vi "RPwithGaGe.vi"(8 "Error In":errorcluster, 10 "Server port":u16=1002, 11 "Server address":string="192.168.1.100") -> (0 "Error Out":errorcluster)   [LabVIEW 2015]
uses:
  Libraries/Red Pitaya/RP Command.ctl
  Libraries/Utilities/Controls/Integrate channel.ctl
  Libraries/GaGe-DAQ/GaGe Digitizer/GaGe Digitizer.lvclass
  Libraries/Red Pitaya/Mode.ctl
  Libraries/Red Pitaya/Red Pitaya Parameters.ctl
panel:
  out "Idot detected":bool
  out "Magnet current":waveform(dbl)(graph)
  in  "Controls":enum32{"Basic", "Advanced"}(tab)
  in  "Idot \ncalibration":dbl=-137722.0
  in  "Parameters":T1={"Ranges"=[1.12291, 20.0], "Output frequency 1"=50000.0, "Output frequency 2"=50000.0, "Trigger offset"=-2000000, "Post-trigger samples"=5767168, "Desimation rate"=64} {"Post-trigger samples" format="0x%x (%d)"; "Trigger offset" format="0x%x (%d)"; "Output frequency 2" format="%#_6p"; "Output frequency 1" format="%#_6p"; "Ranges" format="%#_12g"}
  out "CPU Temperature":dbl(slide)=48.847186279148 scale=0.0..100.0
  out "Current min/max":cluster{"Max":dbl, "Min":dbl}
  in  "Offset duration":dbl=0.95
  in  "Ch to \nintegrate":i32
  in  "Trigger pos acuracy":i32=2
  in  "Signal bits":i32=16
  in  "Read Temperature":bool=TRUE
  in  "Read trigger":bool=TRUE
  in  "Start server":bool
  in  "FPGA Logic":enum16{"Digitizer", "Fast Digitizer"}(ring)
  in  "Auto-save file":bool=TRUE
  in  "Samples to read":u64=67108864 format="0x%x (%d)"
  in  "Record":bool
  out "Server  output":string
  out "Temperature Chart":dbl(graph)=48.847186279148
  out "bytes written":i32=8
  in  "Status":bool
  out "Status response":u32=1
  out "element":u32
  in  "Status offset":u64=8 format="%x"
  out "Record start pos":u32=1
  out "x-y":u32=4294967295
  out "Phase increment 2":u64=1717987
  out "Phase increment 1":u64=1717987
  in  "Process Stop Button":bool
  in  "Read":bool
  in  "Read subset":bool
  out "Data File  Path":path
  out "Trigger state":bool
  in  "Trigger":bool
  in  "Arm":bool
  out "Phase  Graph":u32[](graph)
  in  "Mode":T2=enum."Digitizer"
  out "Waveform Graph":waveform(sgl)[](graph)
  in  "Stop Server":bool
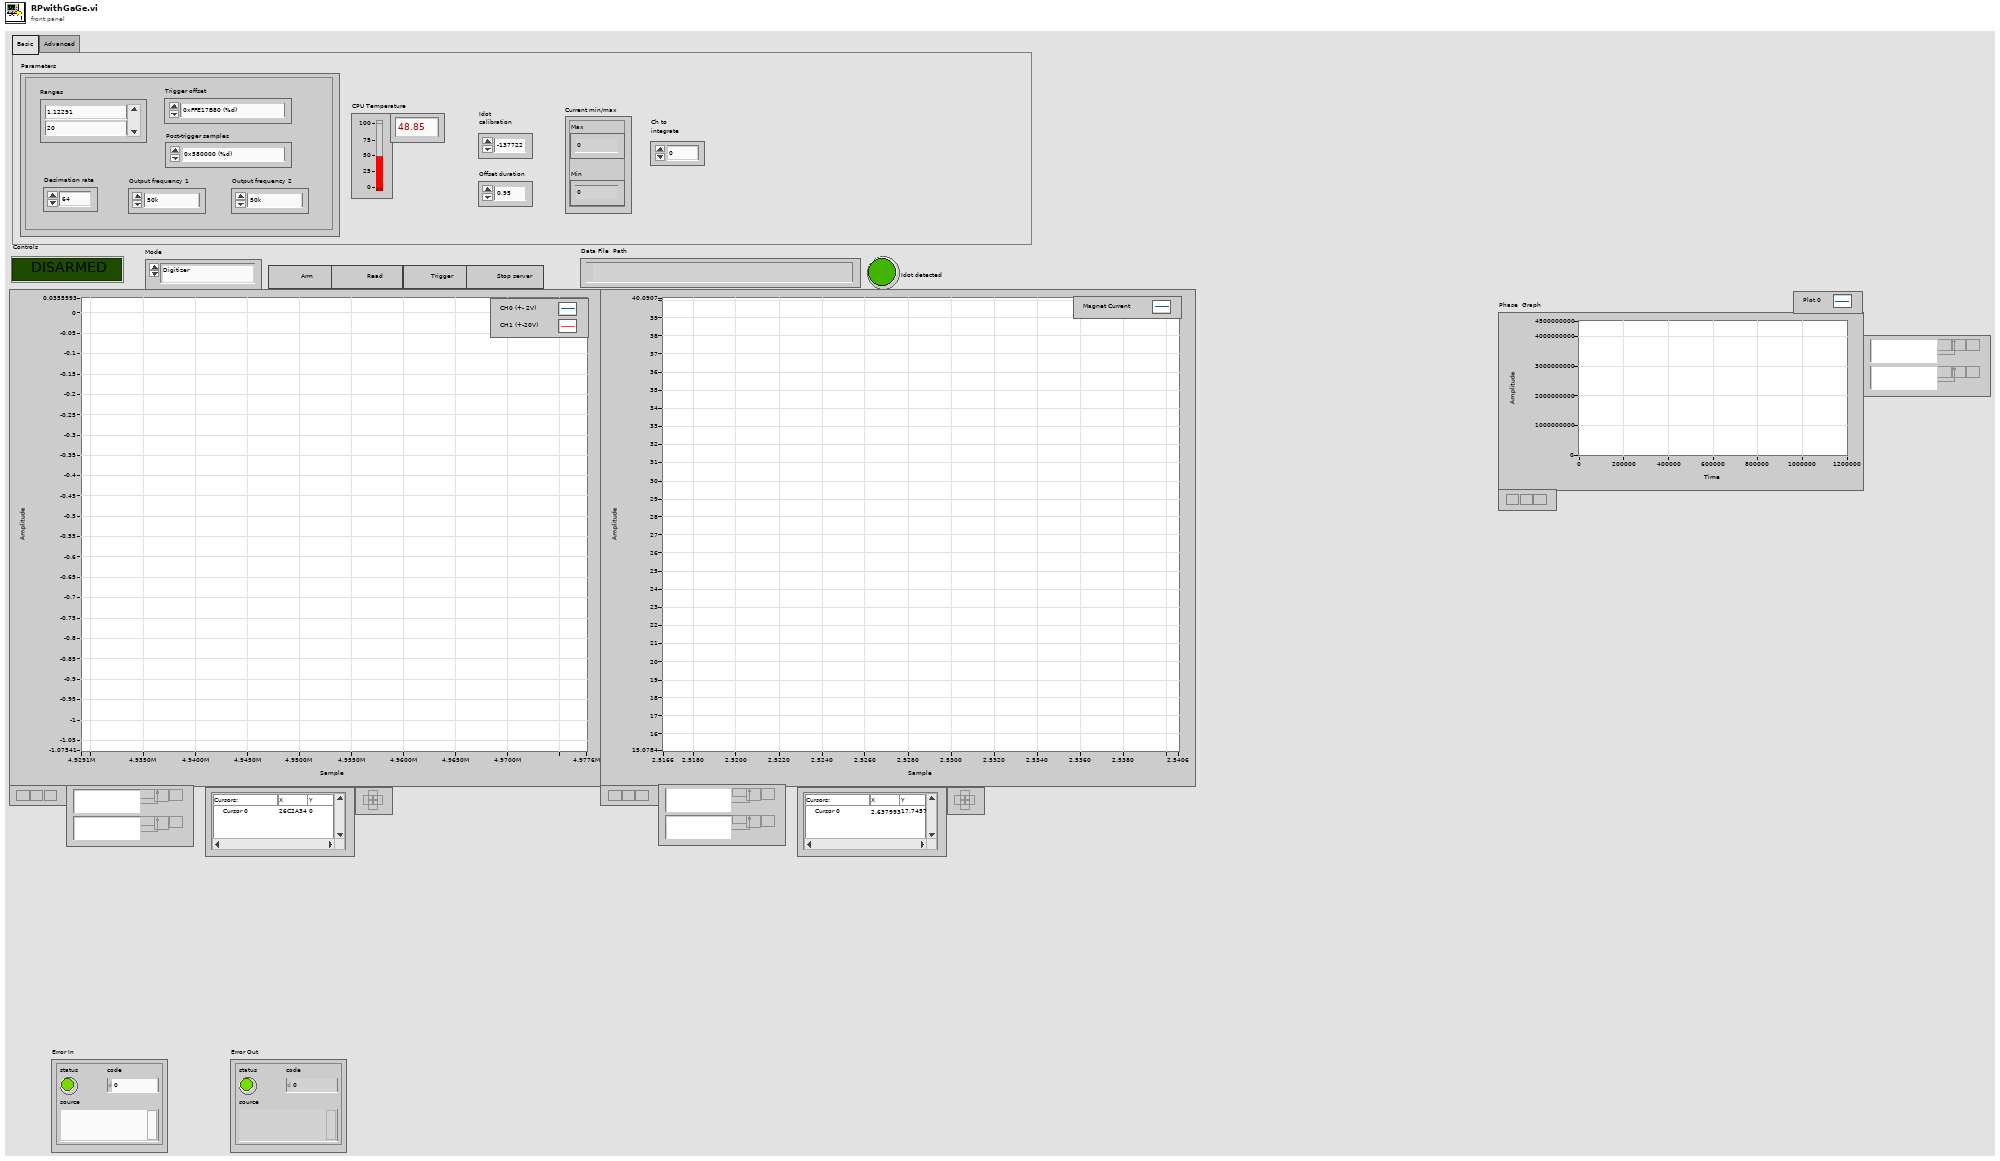
[diagram p1: front panel]
types:
  T1 = typedef "Red Pitaya Parameters.ctl" = cluster{"Ranges":dbl[], "Output frequency 1":dbl, "Output frequency 2":dbl, "Trigger offset":i32, "Post-trigger samples":u64, "Desimation rate":u64}
  T2 = typedef "Mode.ctl" = enum16{"Filter", "Lockin test", "Snapshot test", "Digitizer"}
  T3 = typedef "RP Command.ctl" = enum16{"Set frequency", "Arm and get data", "Stop server", "Get status", "Get temperature", "Set decimation", "Arm", "Software trigger", "Get whole buffer", "Get chunk", "System call", "Get config", "Set config", "Read FIFO", "Play pattern", "Set frequency batch"}
  T4 = enum16{"open", "open or create", "create or replace", "create", "open (read-only)"}
  T5 = typedef "Integrate channel.ctl" = cluster{"Channel":string, "Output name":string, "Factor":dbl, "Start time":dbl, "Duration":dbl}
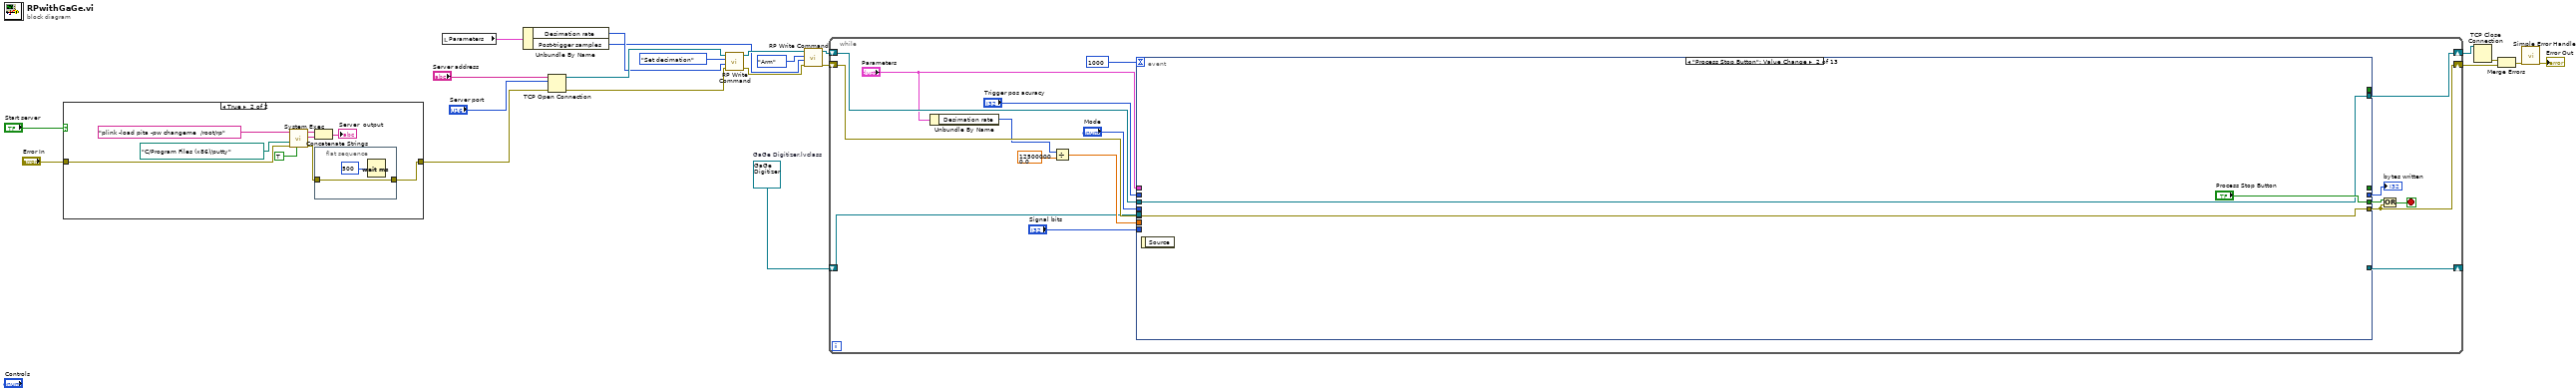
[diagram p0: block diagram]
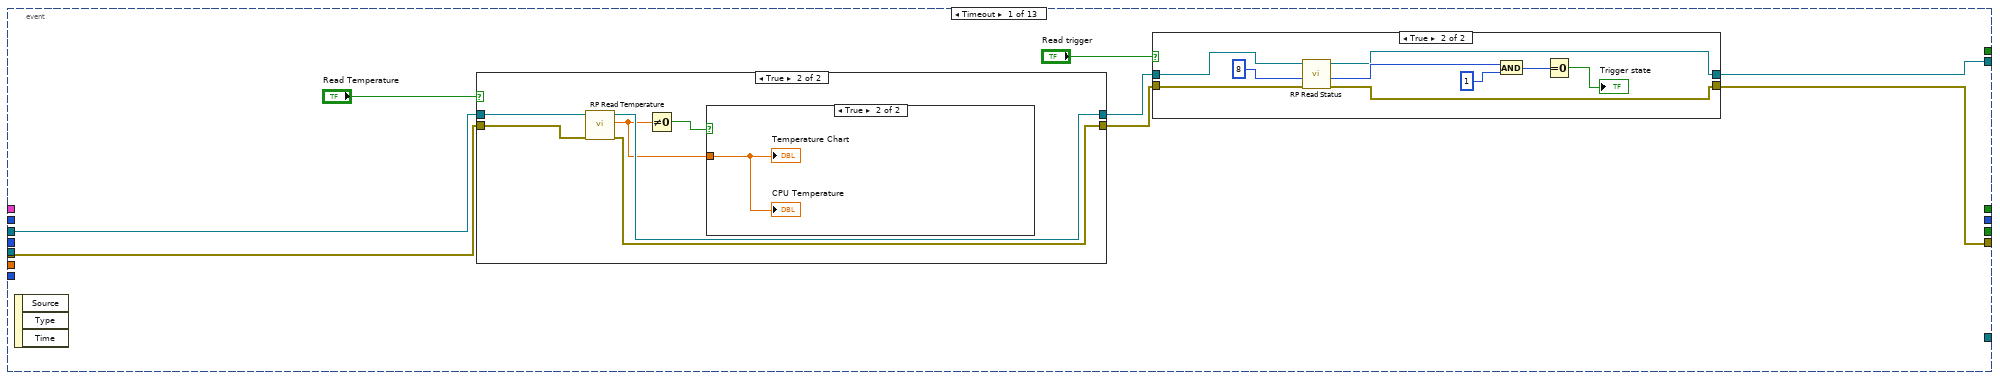
[diagram p3: hidden frame]
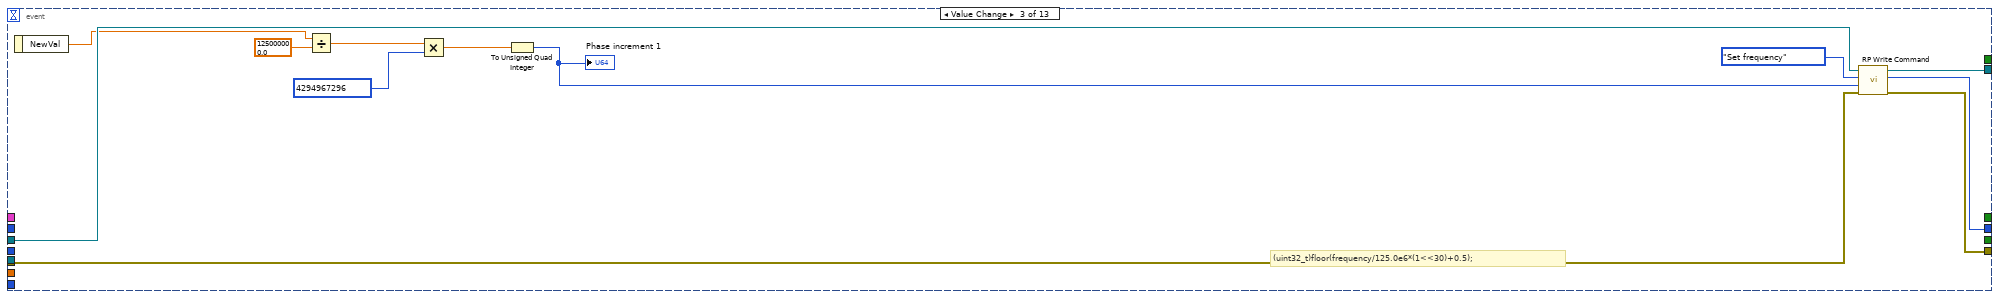
[diagram p7: hidden frame]
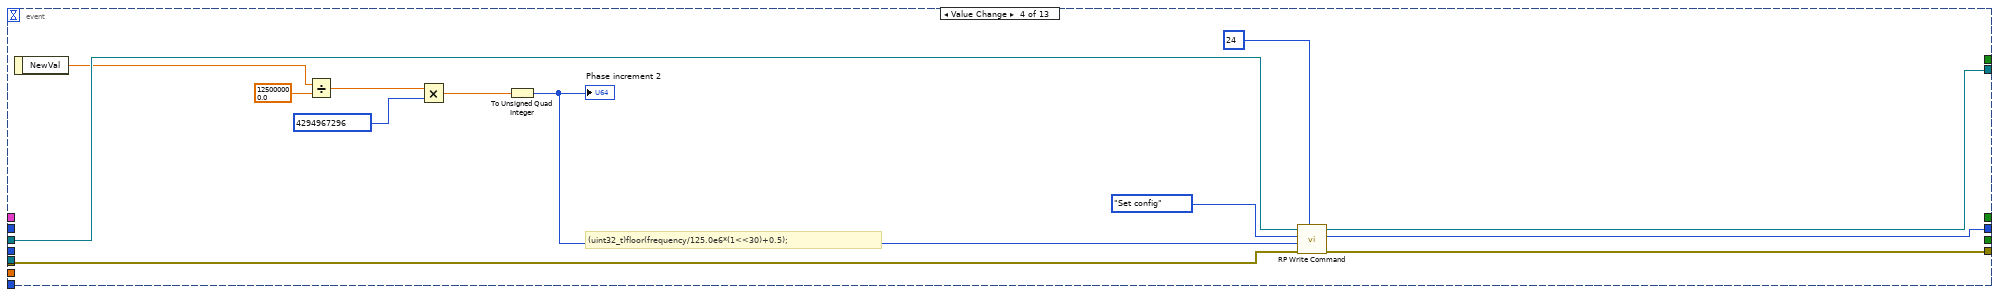
[diagram p8: hidden frame]
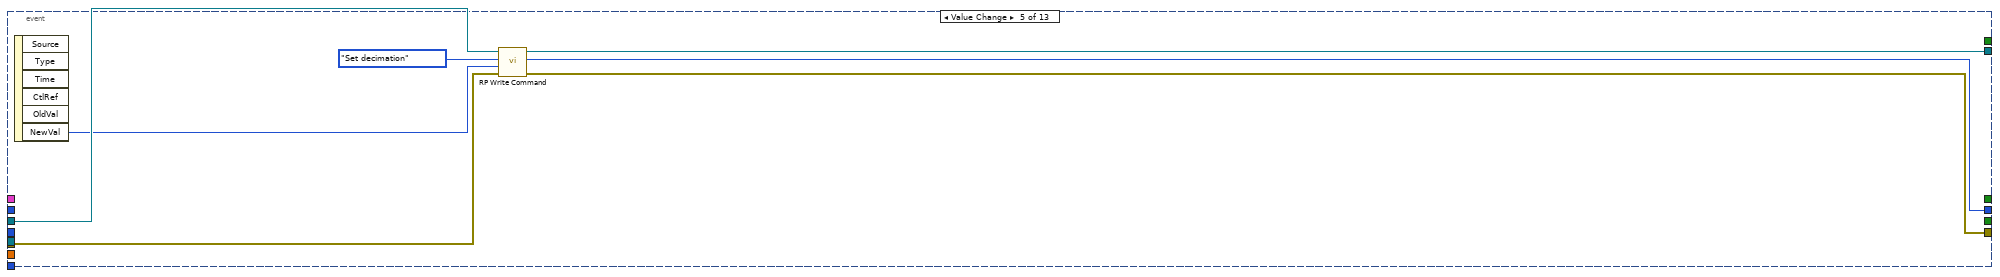
[diagram p9: hidden frame]
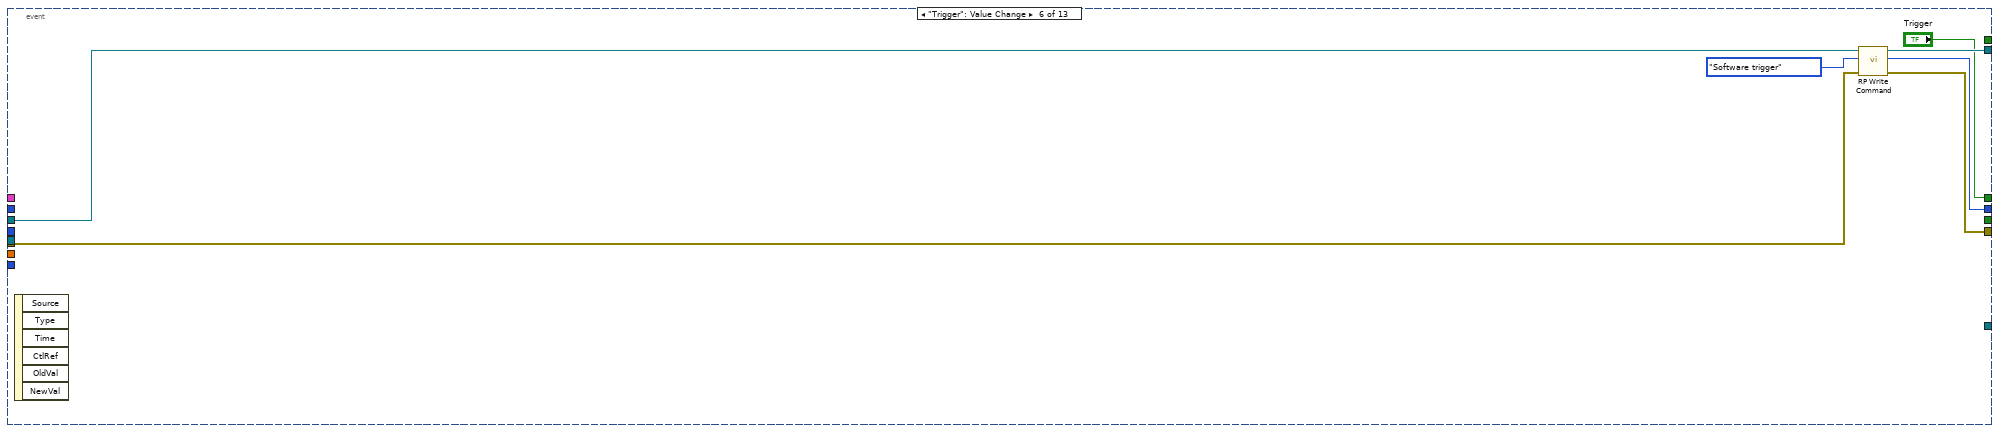
[diagram p10: hidden frame]
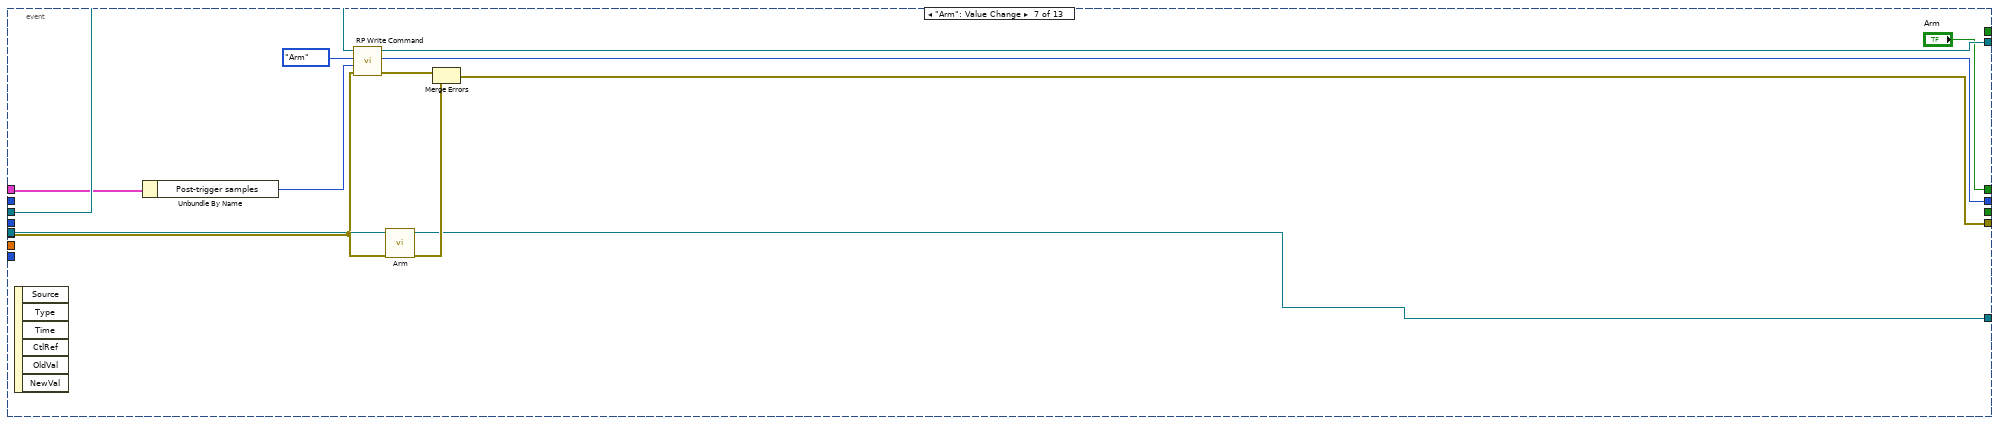
[diagram p11: hidden frame]
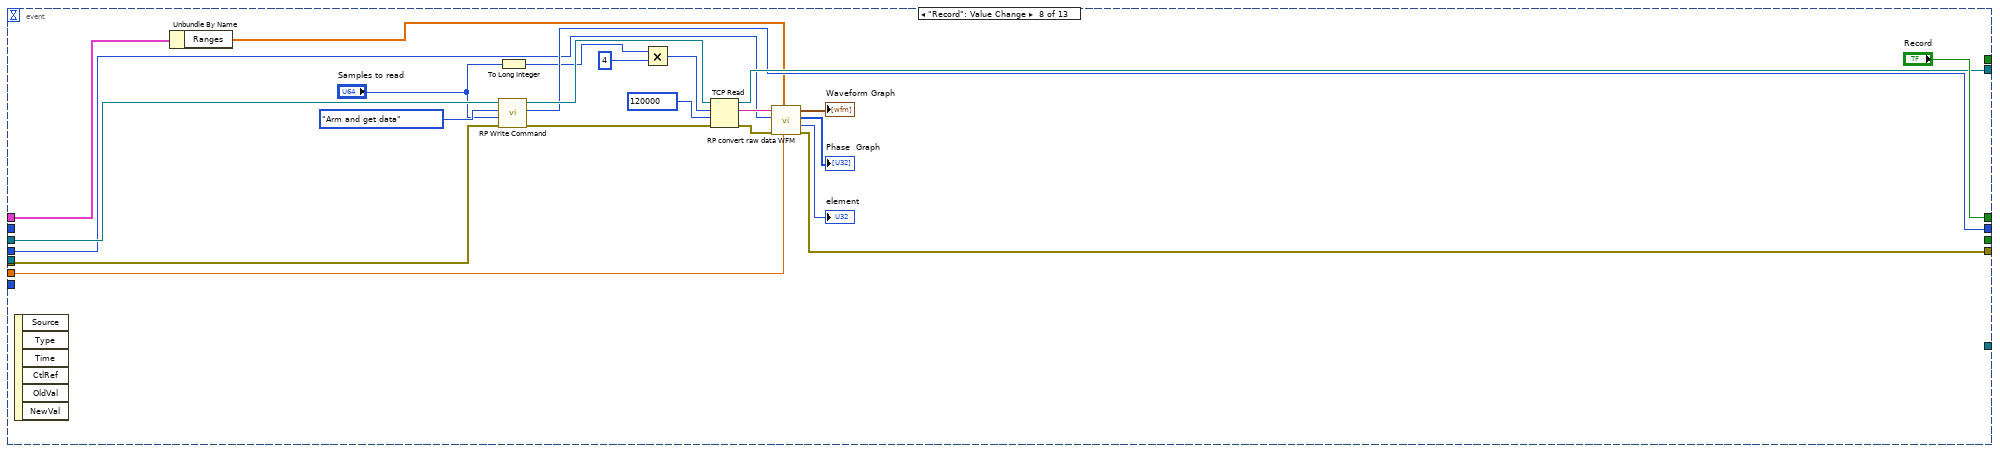
[diagram p12: hidden frame]
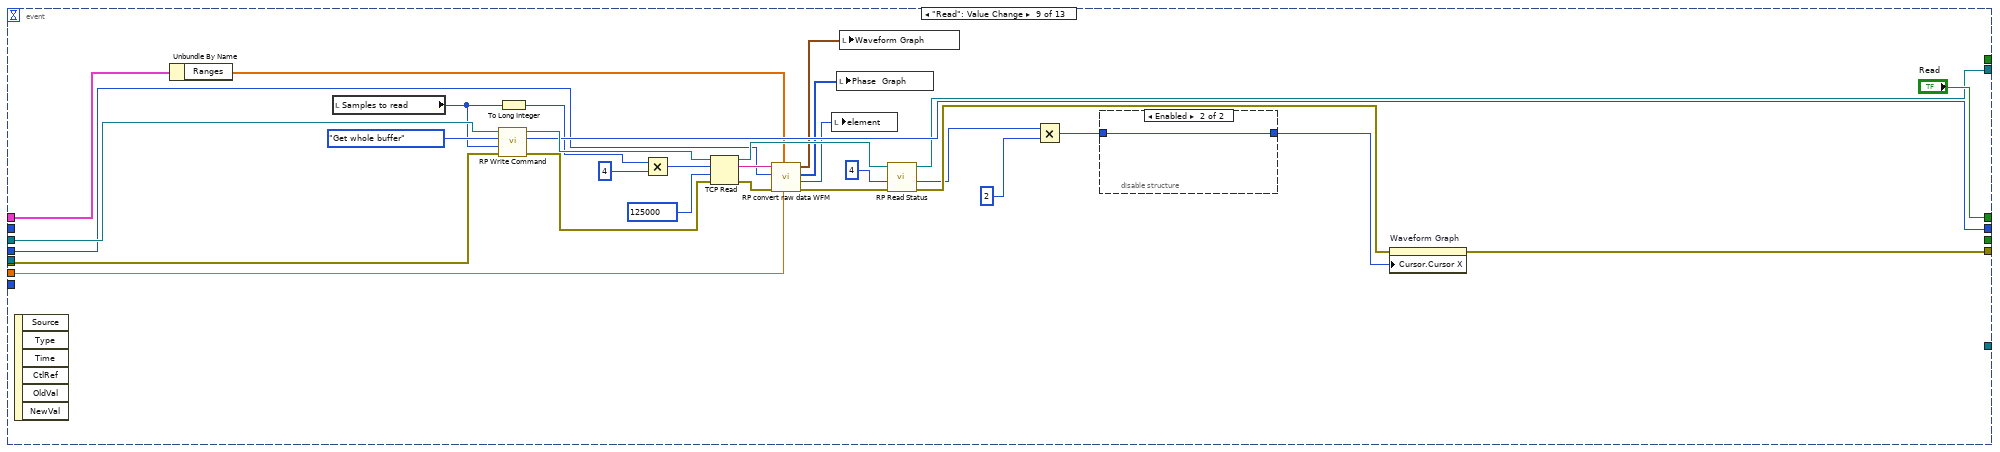
[diagram p13: hidden frame]
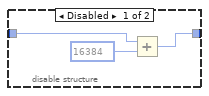
[diagram p14: hidden frame]
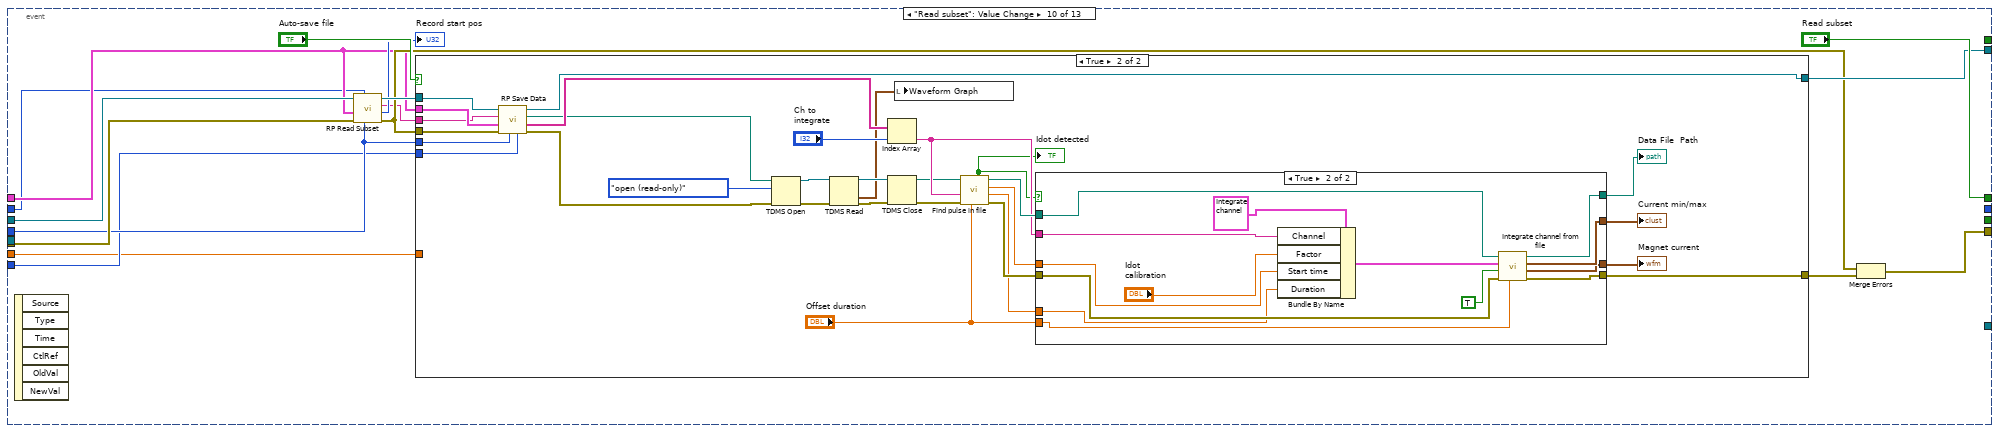
[diagram p15: hidden frame]
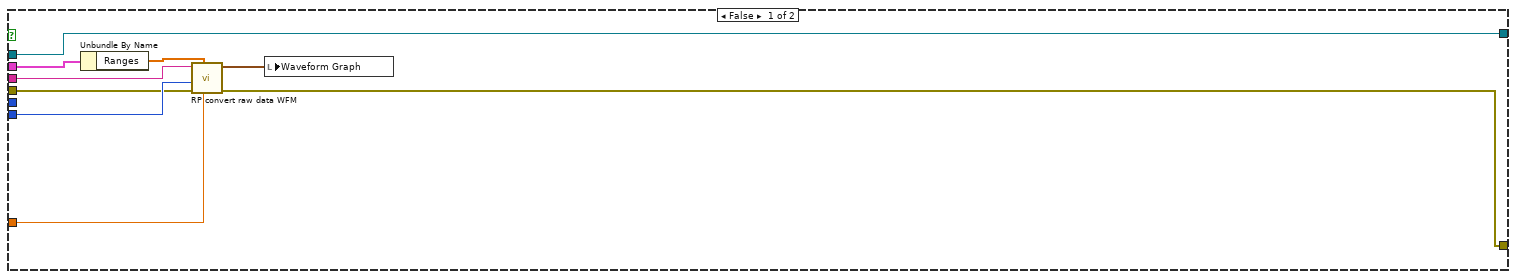
[diagram p16: hidden frame]
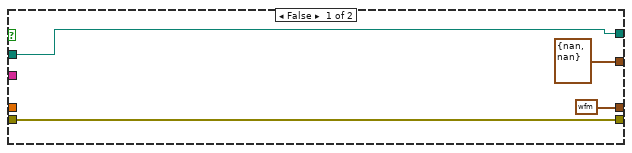
[diagram p17: hidden frame]
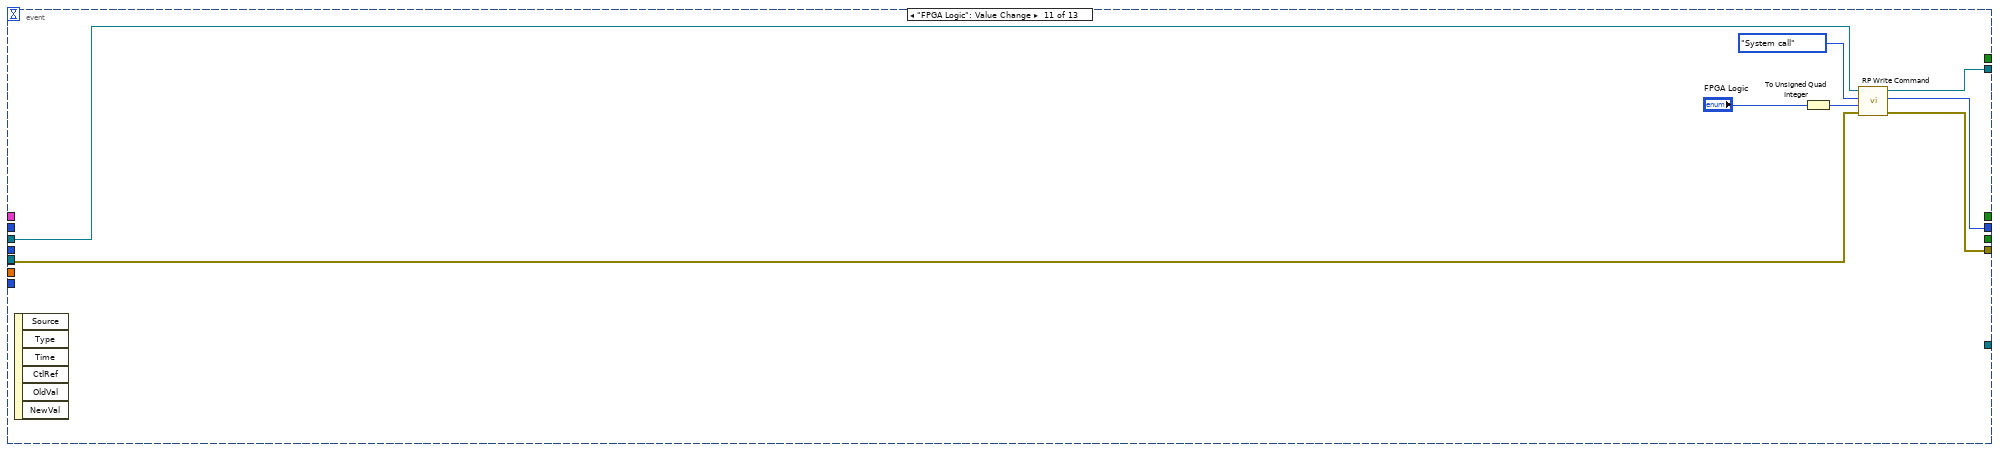
[diagram p18: hidden frame]
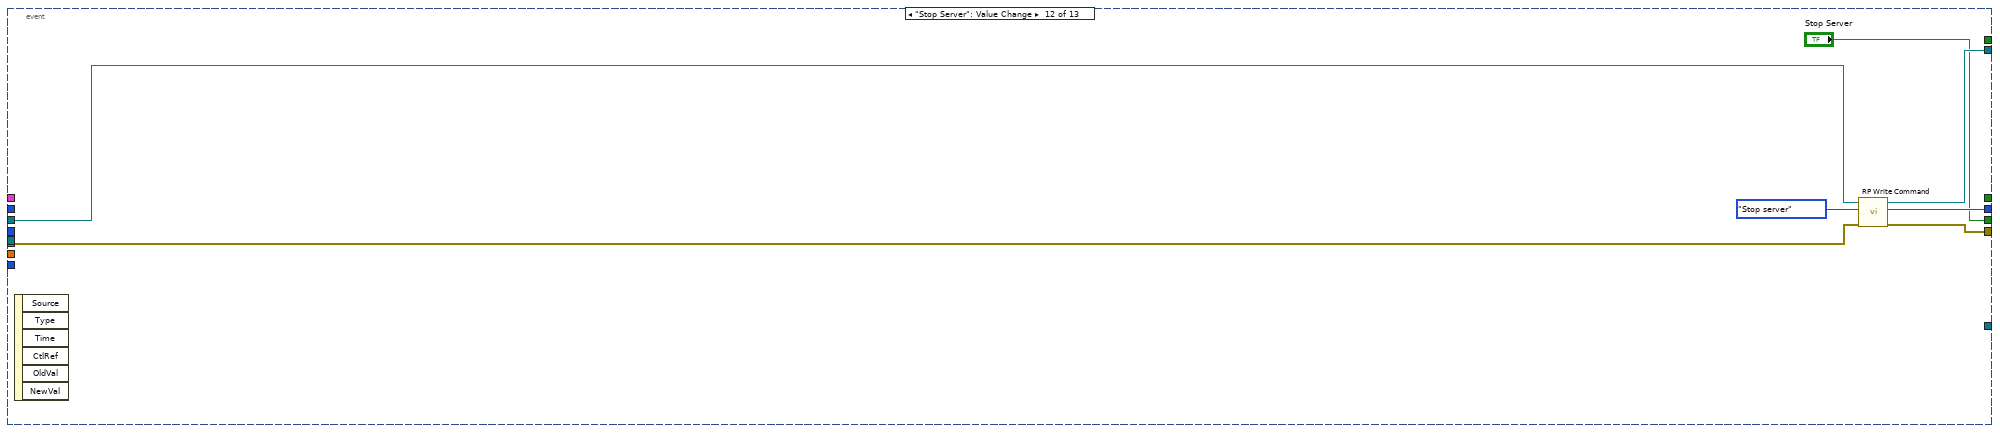
[diagram p19: hidden frame]
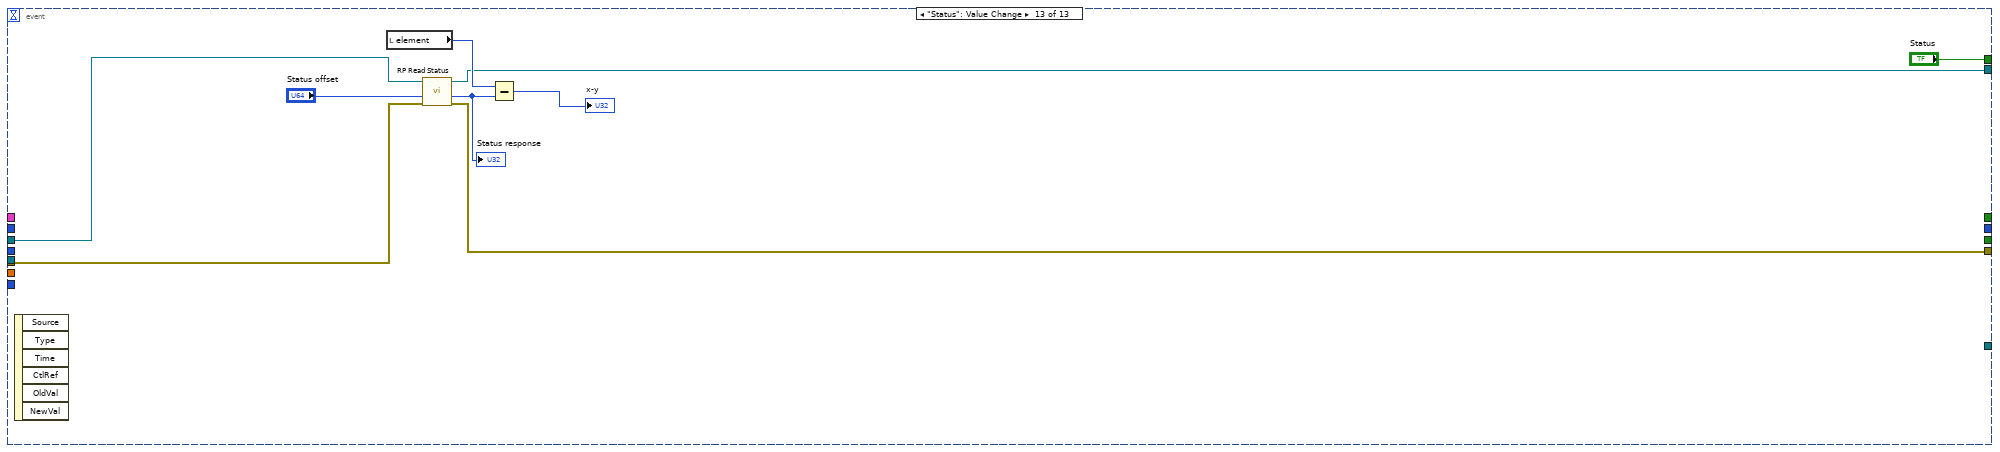
[diagram p20: hidden frame]
diagram:
  w1 = refnum<class "GaGe Digitizer.lvclass"> refnum  # GaGe Digitizer.lvclass
  n1 = case shown="True" "Start server" {
    tunnel: [w23 w24] -> w12
    tunnel: "Error In" -> [w23 w26]
    frame False {
    }
    frame True {
      n2 = call <vilib>:"System Exec.vi"("run minimized? (F)"=TRUE, "error in (no error)"=w26, "working directory"=path "C:/Program Files (x86)/putty", "command line"="plink -load pita -pw changeme  /root/rp") -> ("error out"=w25:errorcluster, "standard error"=w28:string, "standard output"=w32:string)  [unwired: 4 in, 1 out]
      n3 = Concatenate Strings(w32, w28) -> (→"Server  output":string)
      n4 = flat-sequence {
        tunnel: w25 -> [w34]
        tunnel: [w34] -> w24
        frame #0 {
          n5 = Wait (ms)(milliseconds to wait=u32 500) -> ()  [unwired: 1 out]
        }
      }
    }
  }
  n6 = local read "Parameters"() -> (w9:T1)
  n7 = Unbundle By Name(w9) -> ("Desimation rate"=w8:u64, "Post-trigger samples"=w4:u64)
  n8 = TCP Open Connection(address="Server address", remote port or service name="Server port", error in (no error)=w12) -> (connection ID=w10:refnum<k5>, error out=w11:errorcluster)  [unwired: 2 in]
  n9 = call "RP Write Command.vi"("Error In"=w11, "Command payload"=w8, "Command number"=RP_Command."Set decimation", "connection ID"=w10) -> ("Error Out"=w5:errorcluster, "connection ID out"=w6:refnum<k5>)  [unwired: 5 in, 1 out]
  n10 = call "RP Write Command.vi"("Error In"=w5, "Command payload"=w4, "Command number"=RP_Command."Arm", "connection ID"=w6) -> ("Error Out"=w2:errorcluster, "connection ID out"=w3:refnum<k5>)  [unwired: 5 in, 1 out]
  n11 = while {
    shift-right: [w49] -> w18
    shift-left: w3 -> [w50]
    shift-right: [w47] -> w17
    shift-left: w2 -> [w51]
    shift-right: [w35] -> _
    shift-left: w1 -> [w36]
    stop <- w45 stop-if-true
    n12 = Unbundle By Name("Parameters") -> ("Desimation rate"=w39:u64)
    n13 = Divide(x=w39, y=125000000.0) -> (x/y=w37:dbl)
    n14 = event shown="[1] \"Process Stop Button\": Value Change" {
      selector: _ -> [_ _ _ _ _ _ _ _ _ _ _ _ _]
      dyn-events: _ -> [_ _ _ _ _ _ _ _ _ _ _ _ _]
      timeout: 1000 -> [_ _ _ _ _ _ _ _ _ _ _ _ _]
      tunnel: w51 -> [w57 w81 w90 w103 w114 w121 w125 w150 w183 w203 w273 w280 w286]
      tunnel: w50 -> [w58 w80 w89 w102 w113 w120 w134 w153 w186 w202 w272 w278 w282]
      tunnel: [w53 w81 w85 w98 w110 w117 w124 w142 w180 w206 w268 w277 w285] -> w47
      tunnel: [w52 w80 w86 w99 w111 w118 w132 w155 w176 w204 w267 w276 w283] -> w49
      tunnel: [_ "Process Stop Button" _ _ _ _ _ _ _ _ _ "Stop Server" _] -> w46
      tunnel: [_ _ _ _ _ _ _ _ _ _ _ _ "Status"] -> _
      tunnel: [_ _ w84 w97 w109 w116 w130 w148 w181 _ w266 w275 _] -> w48
      tunnel: [_ _ _ _ _ "Trigger" "Arm" "Record" "Read" "Read subset" _ _ _] -> _
      tunnel: "Mode" -> [_ _ _ _ _ _ _ w139 w162 w199 _ _ _]
      tunnel: "Parameters" -> [_ _ _ _ _ _ w128 w138 w161 w197 _ _ _]
      tunnel: "Signal bits" -> [_ _ _ _ _ _ _ _ _ w195 _ _ _]
      tunnel: "Trigger pos acuracy" -> [_ _ _ _ _ _ _ _ _ w196 _ _ _]
      tunnel: w37 -> [_ _ _ _ _ _ _ w135 w158 w193 _ _ _]
      tunnel: w36 -> [_ _ _ _ _ _ w126 _ _ _ _ _ _]
      tunnel: [_ _ _ _ _ _ w122 _ _ _ _ _ _] -> w35
      event Timeout {
        n15 = event-data() -> ()  [unwired: 1 in, 3 out]
        n16 = case shown="True" "Read Temperature" {
          tunnel: w58 -> [w72 w77]
          tunnel: w57 -> [w71 w73]
          tunnel: [w72 w76] -> w55
          tunnel: [w71 w74] -> w54
          frame False {
          }
          frame True {
            n17 = call "RP Read Temperature.vi"("Error In"=w73, "connection ID"=w77) -> ("error out"=w74:errorcluster, "Thermometer"=w75:dbl, "connection ID out"=w76:refnum<k5>)  [unwired: 7 in]
            n18 = Not Equal To 0?(x=w75) -> (x != 0?=w78:bool)
            n19 = case shown="True" w78 {
              tunnel: w75 -> [_ w79]
              frame False {
              }
              frame True {
                "CPU Temperature" <- w79
                "Temperature Chart" <- w79
              }
            }
          }
        }
        n20 = case shown="True" "Read trigger" {
          tunnel: w55 -> [w60 w69]
          tunnel: w54 -> [w61 w70]
          tunnel: [w61 w65] -> w53
          tunnel: [w60 w62] -> w52
          frame False {
          }
          frame True {
            n21 = call "RP Read Status.vi"("Error In"=w70, "Status offset"=u64 8, "connection ID"=w69) -> ("Error Out"=w65:errorcluster, "Status response"=w67:u32, "connection ID out"=w62:refnum<k5>)  [unwired: 6 in]
            n22 = And(x=w67, y=u32 1) -> (x .and. y?=w64:u32)
            n23 = Equal To 0?(x=w64) -> (x = 0?=→"Trigger state":bool)
          }
        }
      }
      event "Process Stop Button": Value Change {
        n24 = event-data() -> ()  [unwired: 1 in, 1 out]
      }
      event Value Change {
        # "(uint32_t)floor(frequency/125.0e6*(1<<30)+0.5);"
        n25 = event-data() -> ("NewVal"=w83:dbl)  [unwired: 1 in]
        n26 = Divide(x=w83, y=125000000.0) -> (x/y=w92:dbl)
        n27 = Multiply(x=w92, y=i64 4294967296) -> (x*y=w91:dbl)
        n28 = To Unsigned Quad Integer(1:w91) -> (0:w87:u64)
        "Phase increment 1" <- w87
        n29 = call "RP Write Command.vi"("Error In"=w90, "Command payload"=w87, "Command number"=RP_Command."Set frequency", "connection ID"=w89) -> ("Error Out"=w85:errorcluster, "bytes written"=w84:i32, "connection ID out"=w86:refnum<k5>)  [unwired: 5 in]
      }
      event Value Change {
        # "(uint32_t)floor(frequency/125.0e6*(1<<30)+0.5);"
        n30 = event-data() -> ("NewVal"=w95:dbl)  [unwired: 1 in]
        n31 = Divide(x=w95, y=125000000.0) -> (x/y=w105:dbl)
        n32 = Multiply(x=w105, y=i64 4294967296) -> (x*y=w104:dbl)
        n33 = To Unsigned Quad Integer(1:w104) -> (0:w100:u64)
        "Phase increment 2" <- w100
        n34 = call "RP Write Command.vi"("Config offset"=u64 24, "Error In"=w103, "Command payload"=w100, "Command number"=RP_Command."Set config", "connection ID"=w102) -> ("Error Out"=w98:errorcluster, "bytes written"=w97:i32, "connection ID out"=w99:refnum<k5>)  [unwired: 4 in]
      }
      event Value Change {
        n35 = event-data() -> ("NewVal"=w108:u64)  [unwired: 1 in, 5 out]
        n36 = call "RP Write Command.vi"("Error In"=w114, "Command payload"=w108, "Command number"=RP_Command."Set decimation", "connection ID"=w113) -> ("Error Out"=w110:errorcluster, "bytes written"=w109:i32, "connection ID out"=w111:refnum<k5>)  [unwired: 5 in]
      }
      event "Trigger": Value Change {
        n37 = event-data() -> ()  [unwired: 1 in, 6 out]
        n38 = call "RP Write Command.vi"("Error In"=w121, "Command number"=RP_Command."Software trigger", "connection ID"=w120) -> ("Error Out"=w117:errorcluster, "bytes written"=w116:i32, "connection ID out"=w118:refnum<k5>)  [unwired: 6 in]
      }
      event "Arm": Value Change {
        n39 = event-data() -> ()  [unwired: 1 in, 6 out]
        n40 = Unbundle By Name(w128) -> ("Post-trigger samples"=w127:u64)
        n41 = call "RP Write Command.vi"("Error In"=w125, "Command payload"=w127, "Command number"=RP_Command."Arm", "connection ID"=w134) -> ("Error Out"=w131:errorcluster, "bytes written"=w130:i32, "connection ID out"=w132:refnum<k5>)  [unwired: 5 in]
        n42 = call-dynamic "Arm.vi"("error in (no error)"=w125, "GaGe Digitizer in"=w126) -> ("error out"=w123:errorcluster, "GaGe Digitizer out"=w122:refnum<class "GaGe Digitizer.lvclass">)  [unwired: 8 in]
        n43 = Merge Errors(w131, w123) -> (w124:errorcluster)
      }
      event "Record": Value Change {
        n44 = event-data() -> ()  [unwired: 1 in, 6 out]
        n45 = Unbundle By Name(w138) -> ("Ranges"=w137:dbl[])
        n46 = call "RP Write Command.vi"("Error In"=w150, "Command payload"="Samples to read", "Command number"=RP_Command."Arm and get data", "connection ID"=w153) -> ("Error Out"=w149:errorcluster, "bytes written"=w148:i32, "connection ID out"=w151:refnum<k5>)  [unwired: 5 in]
        n47 = To Long Integer(number="Samples to read") -> (32bit integer=w147:i32)
        n48 = Multiply(x=w147, y=4) -> (x*y=w154:i32)
        n49 = TCP Read(connection ID=w151, bytes to read=w154, error in (no error)=w149, 9:120000 ("timeout ms (25000)")) -> (connection ID out=w155:refnum<k5>, data out=w144:string, error out=w143:errorcluster)  [unwired: 1 in]
        n50 = call "RP convert raw data WFM.vi"("dt"=w135, "Max Volts"=w137, "Error In"=w143, "Format"=w139, "data stream"=w144) -> ("Error Out"=w142:errorcluster, "element"=→"element":u32, "phase out"=→"Phase  Graph":u32[], "Data out"=→"Waveform Graph":waveform(sgl)[])  [unwired: 3 in]
      }
      event "Read": Value Change {
        n51 = event-data() -> ()  [unwired: 1 in, 6 out]
        n52 = Unbundle By Name(w161) -> ("Ranges"=w160:dbl[])
        n53 = local read "Samples to read"() -> (w175:u64)
        n54 = call "RP Write Command.vi"("Error In"=w183, "Command payload"=w175, "Command number"=RP_Command."Get whole buffer", "connection ID"=w186) -> ("Error Out"=w182:errorcluster, "bytes written"=w181:i32, "connection ID out"=w184:refnum<k5>)  [unwired: 5 in]
        n55 = To Long Integer(number=w175) -> (32bit integer=w178:i32)
        n56 = Multiply(x=w178, y=4) -> (x*y=w187:i32)
        n57 = TCP Read(connection ID=w184, bytes to read=w187, error in (no error)=w182, 9:125000 ("timeout ms (25000)")) -> (connection ID out=w177:refnum<k5>, data out=w173:string, error out=w164:errorcluster)  [unwired: 1 in]
        n58 = call "RP convert raw data WFM.vi"("dt"=w158, "Max Volts"=w160, "Error In"=w164, "Format"=w162, "data stream"=w173) -> ("Error Out"=w163:errorcluster, "element"=w171:u32, "phase out"=w172:u32[], "Data out"=w159:waveform(sgl)[])  [unwired: 3 in]
        n59 = local write "element"(w171) -> ()
        n60 = local write "Phase  Graph"(w172) -> ()
        n61 = local write "Waveform Graph"(w159) -> ()
        n62 = call "RP Read Status.vi"("Error In"=w163, "Status offset"=u64 4, "connection ID"=w177) -> ("Error Out"=w169:errorcluster, "Status response"=w168:u32, "connection ID out"=w176:refnum<k5>)  [unwired: 6 in]
        n63 = Multiply(x=w168, y=u32 2) -> (x*y=w166:u32)
        n64 = disable-structure shown="Enabled" {
          disable-tunnel: w166 -> [w191 w192]
          disable-tunnel: [w189 w192] -> w165
          frame Disabled {
            n65 = Add(x=w191, y=16384) -> (x+y=w189:u32)
          }
          frame Enabled {
          }
        }
        n66 = property on="Waveform Graph" class="WFGraph (strict)"(error in=w169, "Cursor.Cursor X"=w165) -> (error out=w180:errorcluster)  [unwired: 1 in, 1 out]
      }
      event "Read subset": Value Change {
        n67 = event-data() -> ()  [unwired: 1 in, 6 out]
        n68 = call "RP Read Subset.vi"("Mode"=w199, "Trigger pos acuracy"=w196, "Error In"=w203, "Parameters"=w197, "connection ID"=w202) -> ("Error Out"=w200:errorcluster, "Record start pos"=→"Record start pos":u32, "Data stream"=w194:string, "connection ID out"=w201:refnum<k5>)  [unwired: 3 in]
        n69 = case shown="True" "Auto-save file" {
          tunnel: w200 -> [w215 w242]
          tunnel: w194 -> [w213 w245]
          tunnel: [w214 w239] -> w205
          tunnel: w201 -> [w217 w247]
          tunnel: [w217 w243] -> w204
          tunnel: w197 -> [w212 w246]
          tunnel: w199 -> [_ w244]
          tunnel: w195 -> [w216 w241]
          tunnel: w193 -> [w209 _]
          frame False {
            n70 = Unbundle By Name(w212) -> ("Ranges"=w211:dbl[])
            n71 = call "RP convert raw data WFM.vi"("dt"=w209, "Max Volts"=w211, "Error In"=w215, "Signal bits"=w216, "data stream"=w213) -> ("Error Out"=w214:errorcluster, "Data out"=w210:waveform(sgl)[])  [unwired: 3 in, 2 out]
            n72 = local write "Waveform Graph"(w210) -> ()
          }
          frame True {
            n73 = call "RP Save Data.vi"("Signal bits"=w241, "Mode"=w244, "Error In"=w242, "Parameters"=w246, "Data stream"=w245, "connection ID"=w247) -> ("Error Out"=w222:errorcluster, "Channel names"=w238:string[], "Data File  Path"=w228:path, "connection ID out"=w243:refnum<k5>)  [unwired: 2 in]
            n74 = TDMS Open(8:w222, 10:T4."open (read-only)" ("operation (0:open)"), 11:w228) -> (0:w226:errorcluster, 3:w227:refnum<k34>)  [unwired: 4 in]
            n75 = TDMS Read(0:w227, 11:w226) -> (4:w224:refnum<k34>, 10:w219:waveform(dbl)[], 15:w225:errorcluster)  [unwired: 6 in, 3 out]
            n76 = Index Array(array=w238, index="Ch to \nintegrate") -> (element=w232:string)
            n77 = TDMS Close(8:w225, 11:w224) -> (0:w221:errorcluster, 3:w220:path)
            n78 = local write "Waveform Graph"(w219) -> ()
            n79 = call "Find pulse in file.vi"("Offset duration"="Offset duration", "Error In"=w221, "Channel"=w232, "File Path Control"=w220) -> ("Error Out"=w233:errorcluster, "duration"=w230:dbl, "Start time"=w231:dbl, "File Path out"=w234:path, "Found"=w218:bool)  [unwired: 3 in]
            "Idot detected" <- w218
            n80 = case shown="True" w218 {
              tunnel: [w251 w265] -> w240
              tunnel: [w248 w264] -> w239
              tunnel: "Offset duration" -> [_ w261]
              tunnel: [cluster{"Max":dbl, "Min":dbl} {"Max"=nan, "Min"=nan} ("Min max") w260] -> w237
              tunnel: [waveform(dbl) {"t0"=timestamp(0 s since 1904-01-01), "dt"=1.0, "Y"=[]} ("Integrated Waveform") w259] -> w236
              tunnel: w234 -> [w251 w258]
              tunnel: w233 -> [w248 w257]
              tunnel: w232 -> [_ w256]
              tunnel: w231 -> [_ w255]
              tunnel: w230 -> [_ w254]
              frame False {
              }
              frame True {
                n81 = Bundle By Name(cluster=T5 {"Channel"="", "Output name"="Magnet Current", "Factor"=1.0, "Start time"=0.0, "Duration"=0.0} ("Integration settings"), "Channel"=w256, "Factor"="Idot \ncalibration", "Start time"=w255, "Duration"=w254) -> (w263:T5)
                n82 = call "Integrate channel from file.vi"("Offset duration"=w261, "Error In"=w257, "Save data"=TRUE, "Integration settings"=w263, "File Path Control"=w258) -> ("Error Out"=w264:errorcluster, "Integrated Waveform"=w259:waveform(dbl), "Min max"=w260:cluster{"Max":dbl, "Min":dbl}, "File Path out"=w265:path)  [unwired: 3 in]
              }
            }
            "Data File  Path" <- w240
            "Current min/max" <- w237
            "Magnet current" <- w236
          }
        }
        n83 = Merge Errors(w200, w205) -> (w206:errorcluster)
      }
      event "FPGA Logic": Value Change {
        n84 = event-data() -> ()  [unwired: 1 in, 6 out]
        n85 = To Unsigned Quad Integer(1:"FPGA Logic") -> (0:w270:u64)
        n86 = call "RP Write Command.vi"("Error In"=w273, "Command payload"=w270, "Command number"=RP_Command."System call", "connection ID"=w272) -> ("Error Out"=w268:errorcluster, "bytes written"=w266:i32, "connection ID out"=w267:refnum<k5>)  [unwired: 5 in]
      }
      event "Stop Server": Value Change {
        n87 = event-data() -> ()  [unwired: 1 in, 6 out]
        n88 = call "RP Write Command.vi"("Error In"=w280, "Command number"=RP_Command."Stop server", "connection ID"=w278) -> ("Error Out"=w277:errorcluster, "bytes written"=w275:i32, "connection ID out"=w276:refnum<k5>)  [unwired: 6 in]
      }
      event "Status": Value Change {
        n89 = event-data() -> ()  [unwired: 1 in, 6 out]
        n90 = local read "element"() -> (w288:u32)
        n91 = call "RP Read Status.vi"("Error In"=w286, "Status offset"="Status offset", "connection ID"=w282) -> ("Error Out"=w285:errorcluster, "Status response"=w284:u32, "connection ID out"=w283:refnum<k5>)  [unwired: 6 in]
        "Status response" <- w284
        n92 = Subtract(x=w288, y=w284) -> (x-y=→"x-y":u32)
      }
    }
    "bytes written" <- w48
    n93 = Or(x=w46, y=w47) -> (x .or. y?=w45:bool)
  }
  n94 = TCP Close Connection(connection ID=w18) -> (error out=w20:errorcluster)  [unwired: 2 in, 1 out]
  n95 = Merge Errors(w20, w17) -> (w19:errorcluster)
  n96 = call <vilib>:"Simple Error Handler.vi"("error in (no error)"=w19) -> ("error out"=→"Error Out":errorcluster)  [unwired: 4 in, 4 out]
